vi "calculate_resistance.vi"(0 "Bare Resistance (MOhm)":dbl, 1 "Live Resistance":dbl, 2 "Solution Conductance \nS/m":dbl, 3 "Sealed Resistance (MOhm)":dbl, 5 "Membrane Thickness (nm)":dbl, 6 "Override":bool, 7 "Desired Pore Size (nm)":dbl, 14 "Applied Voltage (V)":dbl) -> (4 "Boolean":bool, 8 "Target Resistance (MOhm)":dbl, 9 "Capillary Resistance":dbl, 10 "Capillary Diameter (nm)":dbl, 11 "Membrane-Solution Resistivity":dbl, 12 "Pore Resistance":dbl, 13 "Membrane Resistance (MOhm)":dbl, 16 "Target Golovochenko  (MOhm)":dbl)   [LabVIEW 2016]
panel:
  out "Membrane Thickness (m)":dbl
  out "Target Pore Radius (m)":dbl
  out "Capillary Area m2":dbl
  out "R_Access":dbl
  out "R_Cone":dbl
  out "Capillary Diameter (m)":dbl
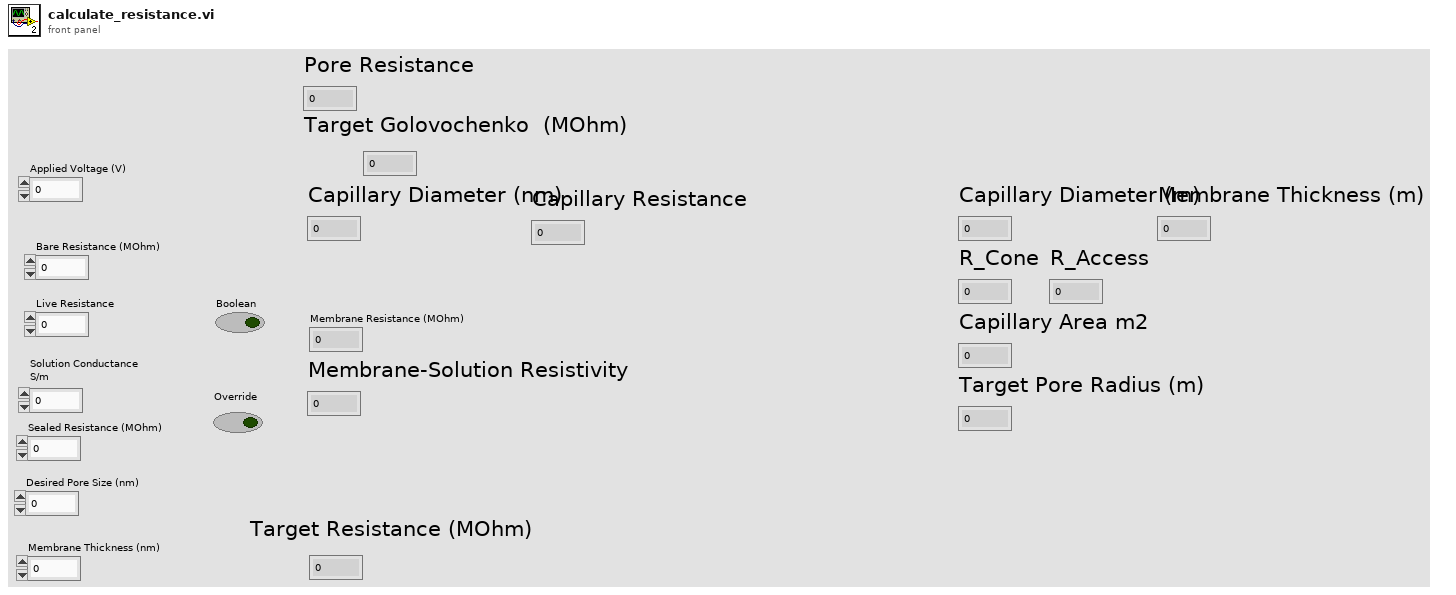
[diagram p1: front panel]
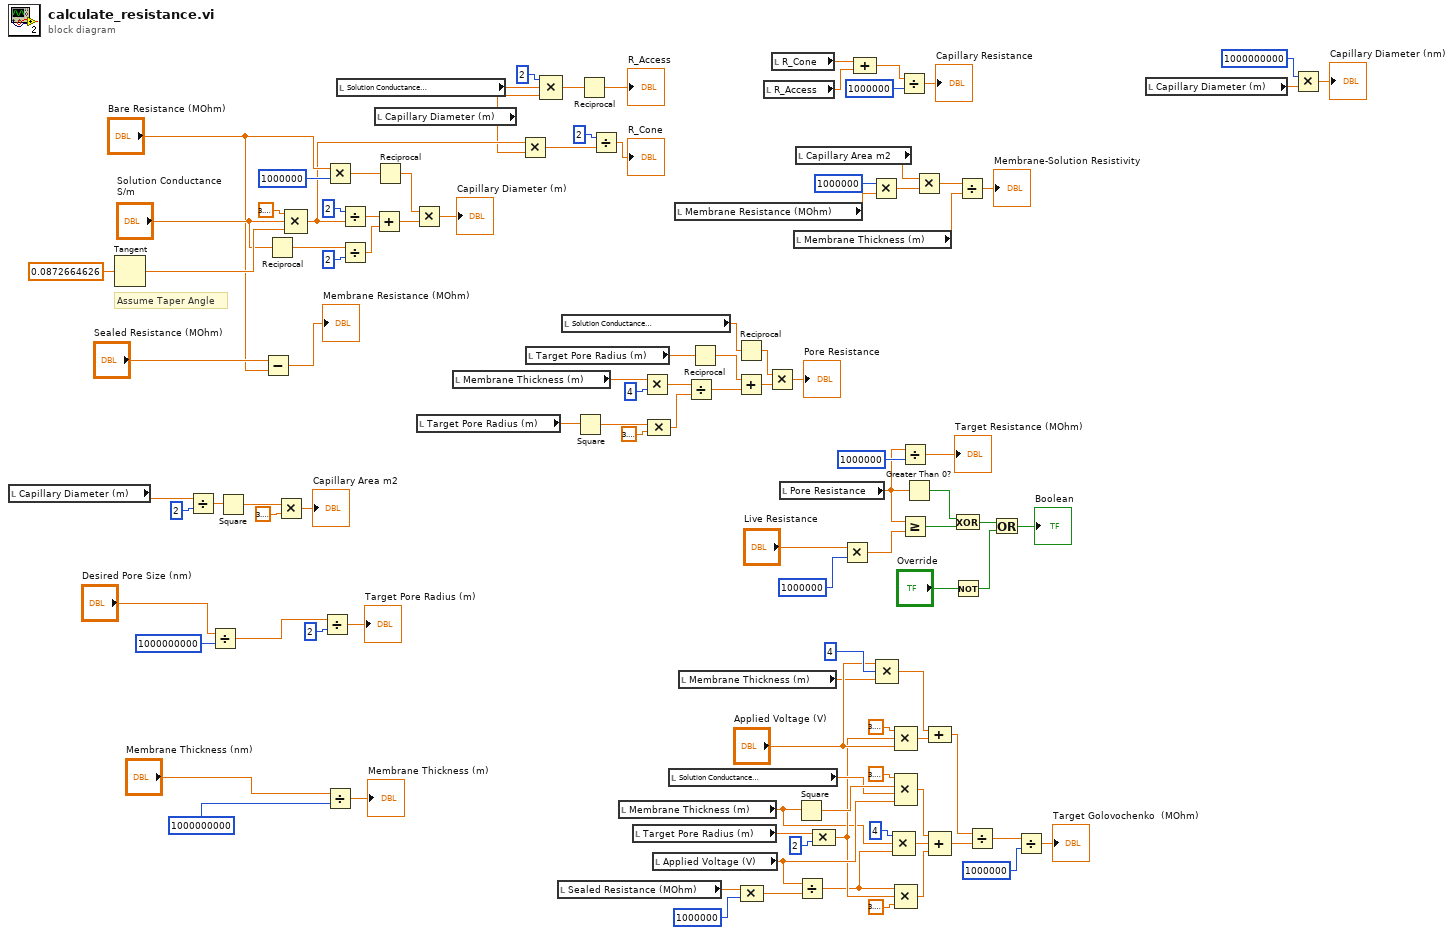
[diagram p0: block diagram]
diagram:
  # "Assume Taper Angle"
  n1 = local read "Capillary Diameter (m)"() -> (w56:dbl)
  n2 = Tangent(1:0.0872664626) -> (0:w105:dbl)
  n3 = Divide(x=w56, y=2) -> (x/y=w88:dbl)
  n4 = Divide(x="Desired Pore Size (nm)", y=1000000000) -> (x/y=w51:dbl)
  n5 = Square(x=w88) -> (x^2=w85:dbl)
  n6 = Subtract(x="Sealed Resistance (MOhm)", y="Bare Resistance (MOhm)") -> (x-y=→"Membrane Resistance (MOhm)":dbl)
  n7 = Reciprocal(x="Solution Conductance \nS/m") -> (1/x=w102:dbl)
  n8 = Multiply(x=w85, y=3.141592653589793) -> (x*y=→"Capillary Area m2":dbl)
  n9 = Compound Arithmetic op=MULTIPLY(3.141592653589793, "Solution Conductance \nS/m", w105) -> (w73:dbl)
  n10 = Divide(x=w51, y=2) -> (x/y=→"Target Pore Radius (m)":dbl)
  n11 = Multiply(x="Bare Resistance (MOhm)", y=1000000) -> (x*y=w92:dbl)
  n12 = Divide(x="Membrane Thickness (nm)", y=1000000000) -> (x/y=→"Membrane Thickness (m)":dbl)
  n13 = local read "Solution Conductance \nS/m"() -> (w65:dbl)
  n14 = Divide(x=2, y=w73) -> (x/y=w71:dbl)
  n15 = Divide(x=w102, y=2) -> (x/y=w101:dbl)
  n16 = Add(x=w71, y=w101) -> (x+y=w96:dbl)
  n17 = local read "Capillary Diameter (m)"() -> (w57:dbl)
  n18 = Reciprocal(x=w92) -> (1/x=w103:dbl)
  n19 = Multiply(x=w103, y=w96) -> (x*y=→"Capillary Diameter (m)":dbl)
  n20 = local read "Target Pore Radius (m)"() -> (w49:dbl)
  n21 = local read "Membrane Thickness (m)"() -> (w42:dbl)
  n22 = Multiply(x=w73, y=w57) -> (x*y=w95:dbl)
  n23 = local read "Target Pore Radius (m)"() -> (w38:dbl)
  n24 = Compound Arithmetic op=MULTIPLY(2, w65, w57) -> (w62:dbl)
  n25 = local read "Sealed Resistance (MOhm)"() -> (w14:dbl)
  n26 = local read "Solution Conductance \nS/m"() -> (w31:dbl)
  n27 = Square(x=w49) -> (x^2=w87:dbl)
  n28 = Reciprocal(x=w62) -> (1/x=→"R_Access":dbl)
  n29 = Divide(x=2, y=w95) -> (x/y=→"R_Cone":dbl)
  n30 = local read "Membrane Thickness (m)"() -> (w9:dbl)
  n31 = local read "Target Pore Radius (m)"() -> (w17:dbl)
  n32 = Multiply(x=w42, y=4) -> (x*y=w40:dbl)
  n33 = Compound Arithmetic op=MULTIPLY(w87, 3.141592653589793) -> (w39:dbl)
  n34 = local read "Applied Voltage (V)"() -> (w19:dbl)
  n35 = local read "Solution Conductance \nS/m"() -> (w20:dbl)
  n36 = local read "Membrane Resistance (MOhm)"() -> (w66:dbl)
  n37 = local read "Membrane Thickness (m)"() -> (w18:dbl)
  n38 = Divide(x=w40, y=w39) -> (x/y=w36:dbl)
  n39 = Reciprocal(x=w38) -> (1/x=w37:dbl)
  n40 = Reciprocal(x=w31) -> (1/x=w30:dbl)
  n41 = Add(x=w37, y=w36) -> (x+y=w35:dbl)
  n42 = Compound Arithmetic op=MULTIPLY(w14, 1000000) -> (w12:dbl)
  n43 = local read "R_Access"() -> (w61:dbl)
  n44 = Multiply(x=w30, y=w35) -> (x*y=→"Pore Resistance":dbl)
  n45 = local read "R_Cone"() -> (w58:dbl)
  n46 = local read "Pore Resistance"() -> (w29:dbl)
  n47 = local read "Membrane Thickness (m)"() -> (w44:dbl)
  n48 = local read "Capillary Area m2"() -> (w45:dbl)
  n49 = Square(x=w9) -> (x^2=w21:dbl)
  n50 = Divide(x=w19, y=w12) -> (x/y=w11:dbl)
  n51 = Compound Arithmetic op=MULTIPLY(w17, 2) -> (w15:dbl)
  n52 = Multiply(x="Live Resistance", y=1000000) -> (x*y=w80:dbl)
  n53 = Compound Arithmetic op=ADD(w58, w61) -> (w77:dbl)
  n54 = Multiply(x=1000000, y=w66) -> (x*y=w67:dbl)
  n55 = Compound Arithmetic op=MULTIPLY("Applied Voltage (V)", 4, w18) -> (w26:dbl)
  n56 = Compound Arithmetic op=MULTIPLY(4, w9, w11) -> (w7:dbl)
  n57 = Compound Arithmetic op=MULTIPLY(3.141592653589793, w15, "Applied Voltage (V)") -> (w25:dbl)
  n58 = Compound Arithmetic op=MULTIPLY(3.141592653589793, w21, w20, w19) -> (w8:dbl)
  n59 = Compound Arithmetic op=MULTIPLY(w11, w15, 3.141592653589793) -> (w6:dbl)
  n60 = Divide(x=w77, y=1000000) -> (x/y=→"Capillary Resistance":dbl)
  n61 = Divide(x=w29, y=1000000) -> (x/y=→"Target Resistance (MOhm)":dbl)
  n62 = Greater Or Equal?(x=w29, y=w80) -> (x >= y?=w109:bool)
  n63 = Greater Than 0?(x=w29) -> (x > 0?=w108:bool)
  n64 = Multiply(x=w45, y=w67) -> (x*y=w83:dbl)
  n65 = Compound Arithmetic op=ADD(w26, w25) -> (w5:dbl)
  n66 = Compound Arithmetic op=ADD(w8, w7, w6) -> (w4:dbl)
  n67 = Exclusive Or(1:w109, 2:w108) -> (0:w99:bool)
  n68 = Not(x="Override") -> (.not. x?=w98:bool)
  n69 = Divide(x=w83, y=w44) -> (x/y=→"Membrane-Solution Resistivity":dbl)
  n70 = Divide(x=w5, y=w4) -> (x/y=w3:dbl)
  n71 = Or(x=w99, y=w98) -> (x .or. y?=→"Boolean":bool)
  n72 = Divide(x=w3, y=1000000) -> (x/y=→"Target Golovochenko  (MOhm)":dbl)
  n73 = local read "Capillary Diameter (m)"() -> (w60:dbl)
  n74 = Multiply(x=1000000000, y=w60) -> (x*y=→"Capillary Diameter (nm)":dbl)
